vi "Set Camera Settings.vi"() -> ()   [LabVIEW 2020, in "examples.lvlib"]
uses:
  examples.lvlib
  6edc065a-5b9d-4876-ad44-0cda83ee0fad.vi
  capture/Stream/Stream.lvclass
  capture/capture.lvlib
  capture/Stream/Get Saturation Parameter Info.vi
  image/image.lvlib
  capture/Stream/Get Brightenss Parameter Info.vi
  capture/Stream/Get Brightenss Parameter.vi
  capture/Stream/Get Contrast Parameter Info.vi
  capture/Stream/Get Contrast Parameter.vi
  capture/Stream/Get Gain Parameter Info.vi
  capture/Stream/Get Powerline Frequency Parameter Info.vi
  capture/Stream/Get Gain Parameter.vi
  capture/Stream/Get Powerline Frequency Parameter.vi
  capture/Stream/Get Zoom Parameter.vi
  image/New Image (ARGB Preallocated).vi
  capture/Stream/Get Backlight Compensation Parameter.vi
  capture/Stream/Get Hue Parameter Info.vi
  capture/Stream/Get Hue Parameter.vi
  capture/Stream/Get Gamma Parameter Info.vi
  capture/Stream/Get Gamma Parameter.vi
  capture/Stream/Get Zoom Parameter Info.vi
  capture/Stream/Get White Balance Parameter Info.vi
  capture/Stream/Get Saturation Parameter.vi
  capture/Stream/Get White Balance Parameter.vi
  capture/Stream/Get Sharpness Parameter.vi
  capture/Stream/Get Focus Parameter Info.vi
  capture/Stream/Get Exposure Parameter Info.vi
  capture/Stream/Get Exposure Parameter.vi
  capture/Stream/Get Focus Parameter.vi
  capture/Stream/Get Backlight Compensation Parameter Info.vi
  capture/Stream/Set Powerline Frequency Parameter.vi
  capture/Stream/Set Hue Parameter.vi
  capture/Stream/Set White Balance Parameter.vi
  capture/Stream/Set Brightenss Parameter.vi
  capture/Stream/Set Zoom Parameter.vi
  capture/Stream/Set Contrast Parameter.vi
  capture/Stream/Set Gain Parameter.vi
  capture/Stream/Set Backlight Compensation Parameter.vi
  capture/Stream/Set Saturation Parameter.vi
  capture/Stream/Set Gamma Parameter.vi
  capture/Stream/Set Focus Parameter.vi
  capture/Stream/Set Sharpness Parameter.vi
  capture/Stream/Set Exposure Parameter.vi
  image/Draw Image to Picture (ARGB).vi
  dec5b208-33d2-3fcd-38b9-acb140bbe53f.vi
panel:
  in  "Hue":i32(slide) scale=-180.0..180.0
  in  "Gamma":i32(slide) scale=90.0..150.0
  in  "Zoom":i32(slide) scale=100.0..400.0
  in  "Whitebalance":i32(slide) scale=2800.0..6500.0
  in  "Sharpness":i32(slide) scale=0.0..100.0
  in  "Saturation":i32(slide) scale=0.0..100.0
  in  "Powerline Frequency":i32(slide) scale=-180.0..180.0
  in  "Gain":i32(slide) scale=0.0..2.0
  in  "Backlight Compensation":i32(slide) scale=0.0..2.0
  in  "Focus":i32(slide) scale=-11.0..-3.0
  in  "Exposure":i32(slide) scale=-11.0..-3.0
  in  "Contrast":i32(slide) scale=0.0..255.0
  in  "Brightness":i32(slide) scale=0.0..255.0
  out "2D Picture":picture
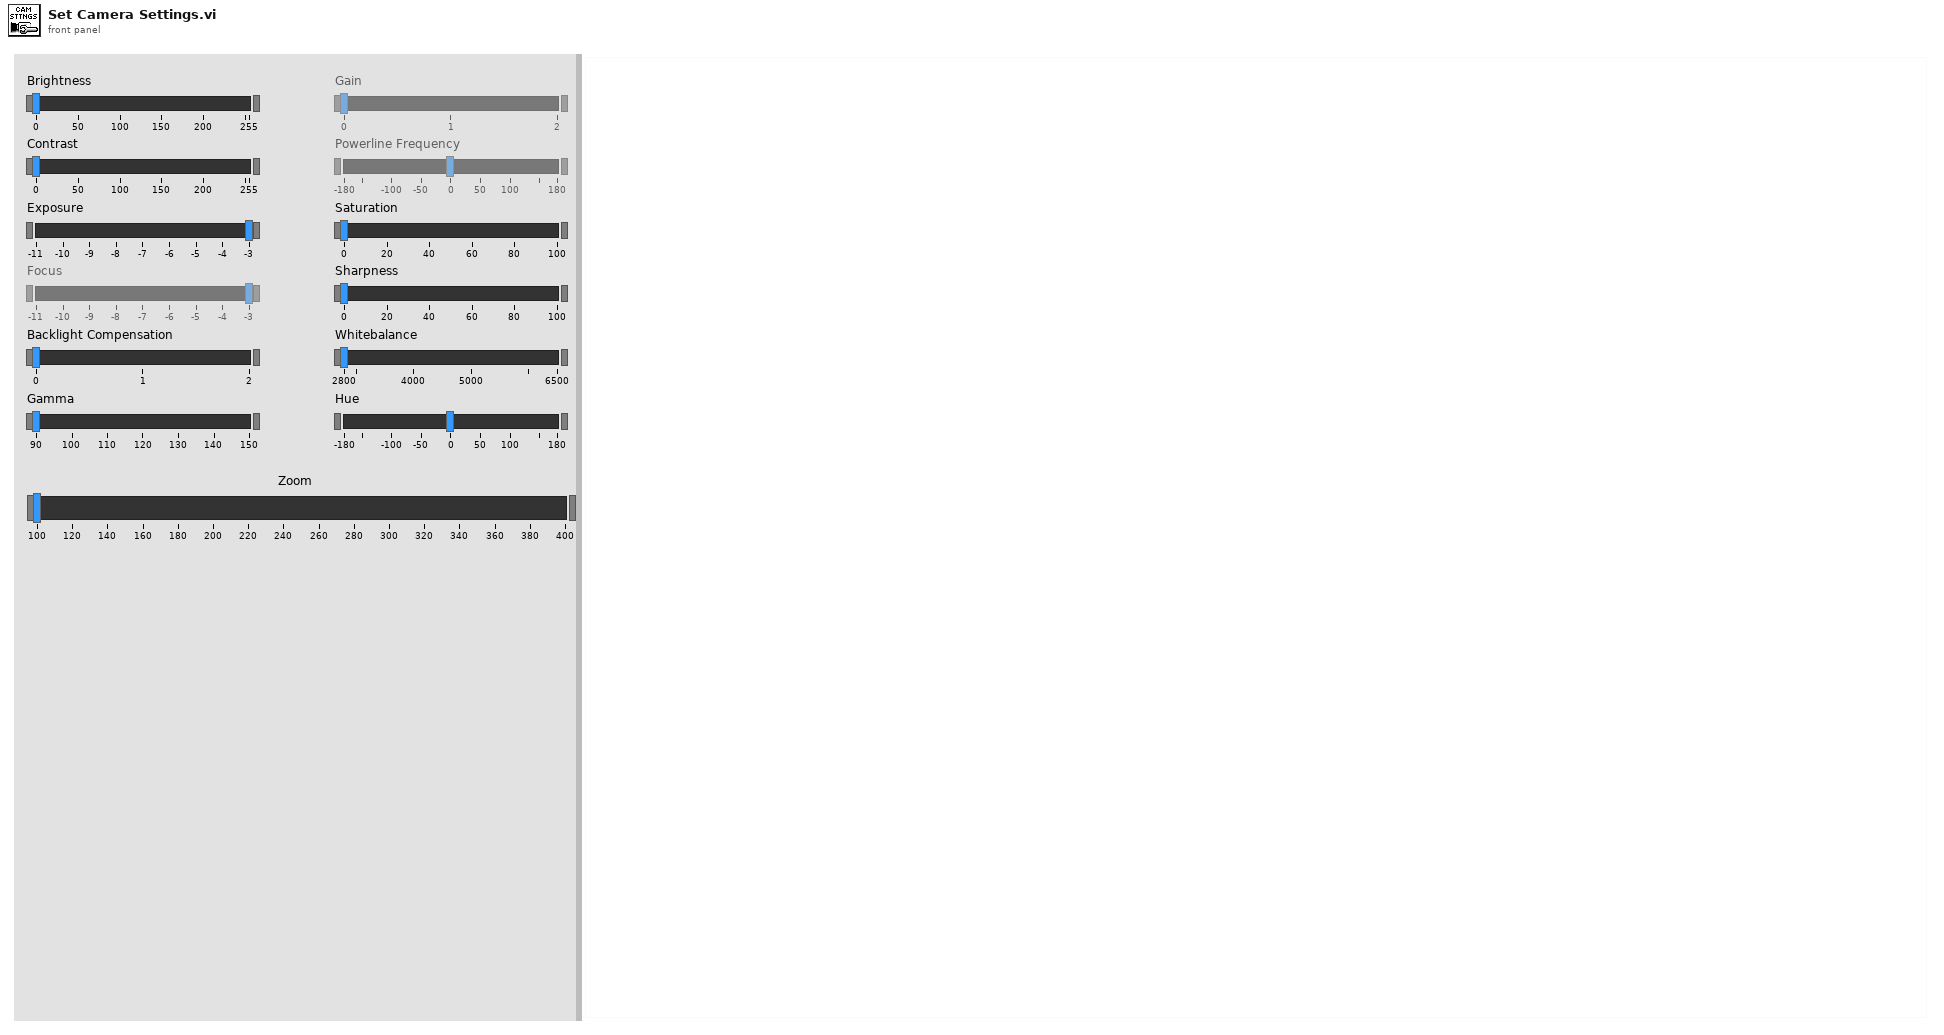
[diagram p1: front panel]
types:
  T1 = enum16{"Brightness", "Contrast", "Exposure", "Focus", "Backlight Compensation", "Gain", "Gamma", "Hue", "Powerline Frequency", "Saturation", "Sharpness", "Whitebalance", "Zoom"}
  T2 = typedef "capture.lvlib/Stream.lvclass/Stream Specification.ctl" = cluster{"Size":T3, "FPS":T4}
  T3 = typedef "common.lvlib/Image Size (Integer).ctl" = cluster{"Width":u16, "Height":u16}
  T4 = typedef "capture.lvlib/Stream.lvclass/Frames per Second.ctl" = cluster{"Numerator":u32, "Denominator":u32}
  T5 = cluster{"ID":string, "Name":string, "Stream Specifications":T2[]}[]
  T6 = cluster{"ID":string, "Name":string, "Stream Specifications":T2[]}
  T7 = enum16{"Brightness", "Contrast", "Exposure", "Focus", "Backlight Compensation", "Gain", "Gamma", "Hue", "Powerline Frequency", "Saturation", "Sharpness", "Whitebalance", "Zoom"}[]
  T8 = enum8{"Enabled", "Disabled", "Disabled and Grayed Out"}
  T9 = typedef "capture.lvlib/Stream.lvclass/Camera Parameter Information.ctl" = cluster{"Is Supported":bool, "Max":i32, "Min":i32, "Step":i32, "Default":i32}
  T10 = typedef "image.lvlib/ARGB Image.ctl" = refnum<data-value>
  T11 = typedef "image.lvlib/Image Draw Offset.ctl" = cluster{"Left":i16, "Top":i16}
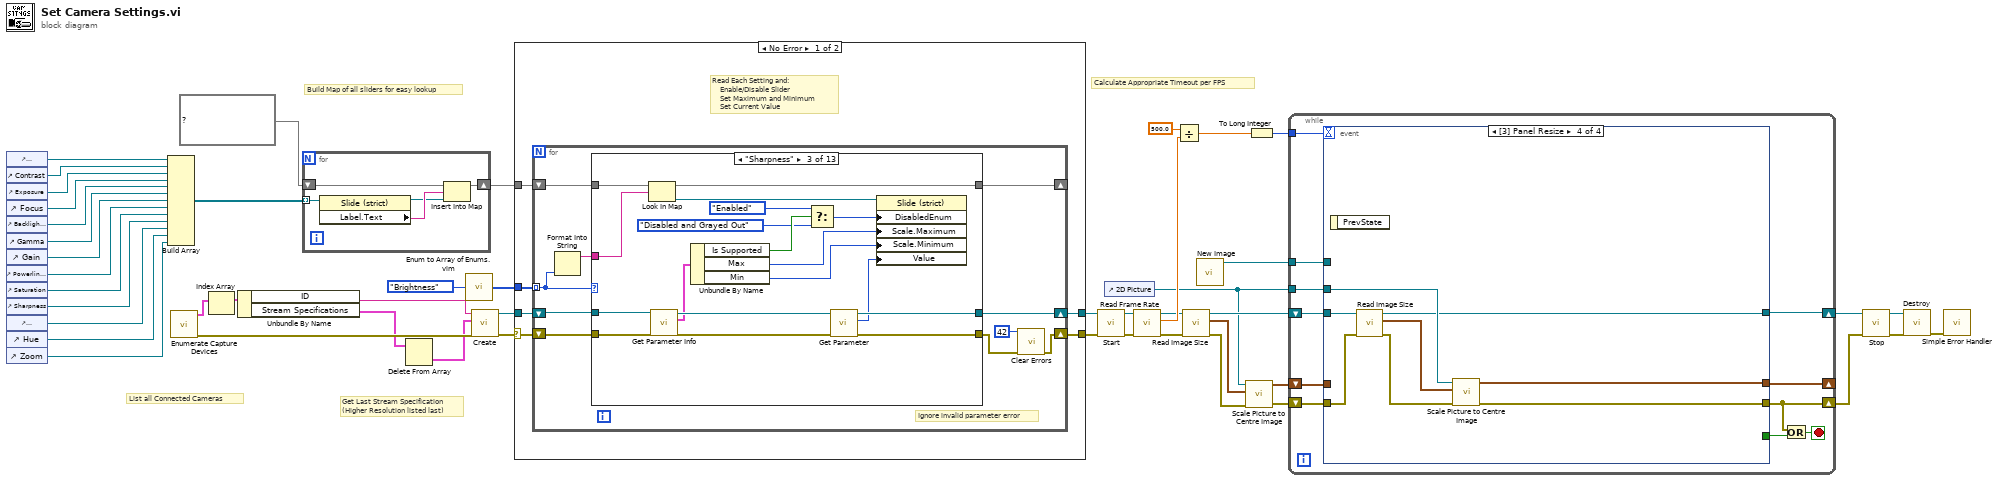
[diagram p0: block diagram]
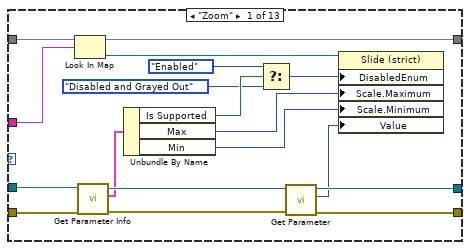
[diagram p2: hidden frame]
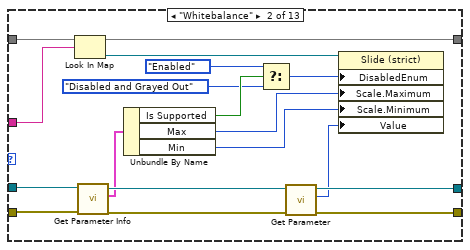
[diagram p3: hidden frame]
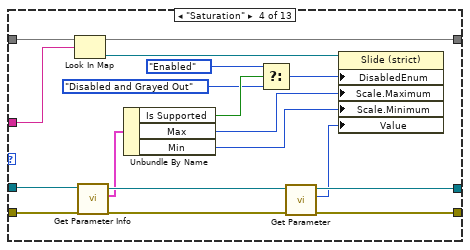
[diagram p4: hidden frame]
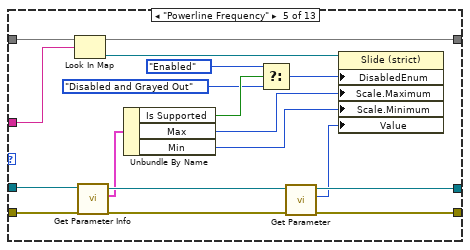
[diagram p5: hidden frame]
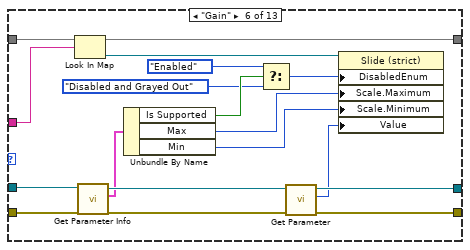
[diagram p6: hidden frame]
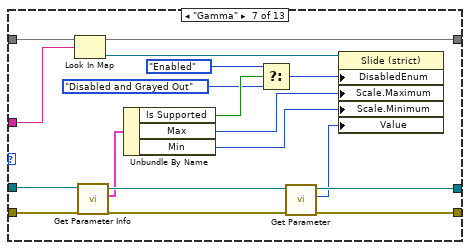
[diagram p7: hidden frame]
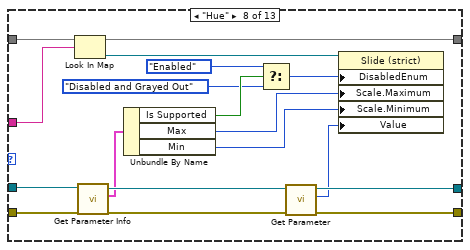
[diagram p8: hidden frame]
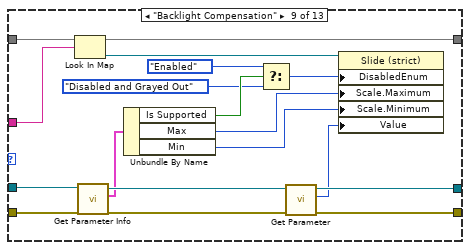
[diagram p9: hidden frame]
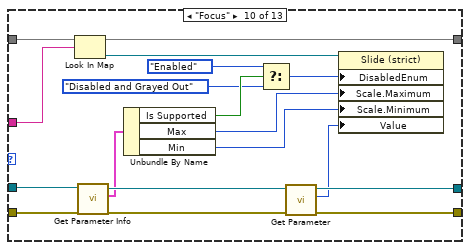
[diagram p10: hidden frame]
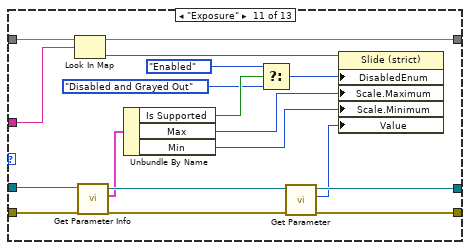
[diagram p11: hidden frame]
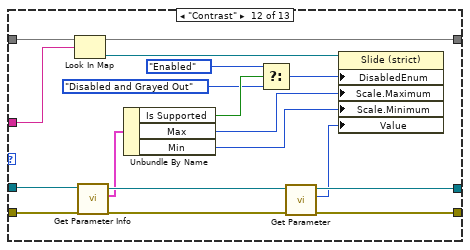
[diagram p12: hidden frame]
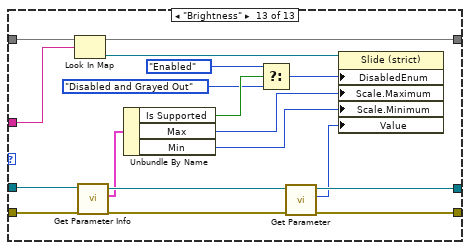
[diagram p13: hidden frame]
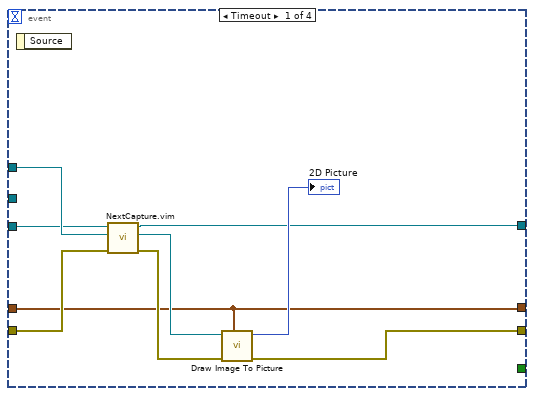
[diagram p15: hidden frame]
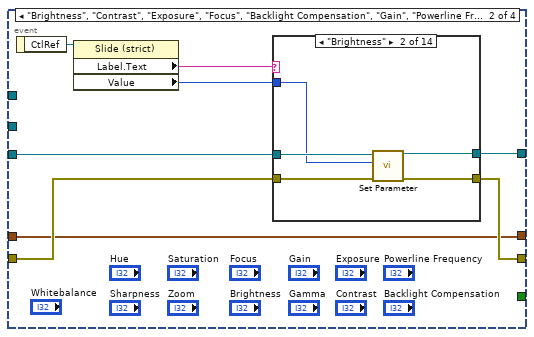
[diagram p16: hidden frame]
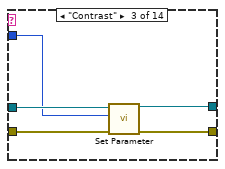
[diagram p18: hidden frame]
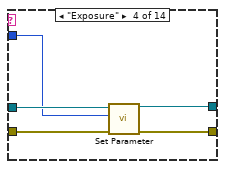
[diagram p19: hidden frame]
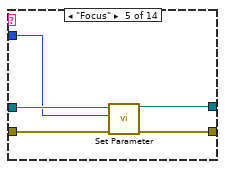
[diagram p20: hidden frame]
diagram:
  # "Calculate Appropriate Timeout per FPS"
  # "Build Map of all sliders for easy lookup"
  # "Get Last Stream Specification\n(Higher Resolution listed last)"
  # "List all Connected Cameras"
  n1 = control-ref of="Brightness"() -> (w40:refnum<vi>)
  n2 = control-ref of="Contrast"() -> (w39:refnum<vi>)
  n3 = control-ref of="Exposure"() -> (w38:refnum<vi>)
  n4 = control-ref of="Focus"() -> (w37:refnum<vi>)
  n5 = control-ref of="Backlight Compensation"() -> (w36:refnum<vi>)
  n6 = control-ref of="Gamma"() -> (w35:refnum<vi>)
  n7 = control-ref of="Gain"() -> (w34:refnum<vi>)
  n8 = control-ref of="Powerline Frequency"() -> (w33:refnum<vi>)
  n9 = control-ref of="Saturation"() -> (w32:refnum<vi>)
  n10 = control-ref of="Sharpness"() -> (w31:refnum<vi>)
  n11 = control-ref of="Whitebalance"() -> (w30:refnum<vi>)
  n12 = control-ref of="Hue"() -> (w29:refnum<vi>)
  n13 = control-ref of="Zoom"() -> (w28:refnum<vi>)
  n14 = Build Array(w40, w39, w38, w37, w36, w35, w34, w33, w32, w31, w30, w29, w28) -> (w27:refnum<vi>[])
  n15 = call "Enumerate Capture Devices.vi"() -> ("error out"=w42:errorcluster, "Devices"=w45:T5)  [unwired: 10 in]
  n16 = Index Array(array=w45) -> (element=w44:T6)  [unwired: 1 in]
  n17 = Unbundle By Name(w44) -> ("ID"=w43:string, "Stream Specifications"=w10:T2[])
  n18 = for {
    tunnel: w27 -> [w53] mode=indexing
    shift-right: [w49] -> w25
    shift-left: map{string, refnum<vi>} {} ("map in") -> [w50]
    n19 = property class="Slide (strict)"(reference=w53) -> (reference out=w51:refnum<vi>, "Label.Text"=w52:string)  [unwired: 1 in, 1 out]
    n20 = Insert Into Map(map in=w50, key=w52, value=w51) -> (map out=w49:map{string, refnum<vi>})  [unwired: 2 out]
  }
  n21 = Delete From Array(array=w10) -> (deleted portion=w41:T2)  [unwired: 2 in, 1 out]
  n22 = call "Enum to Array of Enums.vim"("enum"=T1."Brightness") -> ("array of enums"=w47:T7)
  n23 = call "Create.vi"("error in (no error)"=w42, "Desired Stream Specification"=w41, "Device ID"=w43) -> ("error out"=w9:errorcluster, "Stream"=w46:refnum<class "Stream.lvclass">)  [unwired: 7 in]
  n24 = case shown="No Error" w9 {
    selector: w9 -> [w55 w291]
    tunnel: w47 -> [w59 _]
    tunnel: w46 -> [w58 w292]
    tunnel: w25 -> [w57 _]
    tunnel: [w56 w292] -> w21
    tunnel: [w54 w291] -> w8
    frame No Error {
      # "Read Each Setting and:\n    Enable/Disable Slider\n    Set Maximum and Minimum\n    Set Current Value"
      n25 = for {
        tunnel: w59 -> [w61] mode=indexing
        shift-right: [w68] -> w56
        shift-left: w58 -> [w69]
        shift-right: [w66] -> _
        shift-left: w57 -> [w67]
        shift-right: [w62] -> w54
        shift-left: w55 -> [w65]
        # "Ignore invalid parameter error"
        n26 = Format Into String(w61) -> (resulting string=w60:string)  [unwired: 3 in, 1 out]
        n27 = case shown="\"Sharpness\"" w61 {
          tunnel: w69 -> [w86 w103 w120 w137 w154 w171 w188 w205 w222 w239 w256 w273 w290]
          tunnel: [w84 w100 w117 w134 w151 w168 w185 w202 w219 w236 w253 w270 w287] -> w68
          tunnel: w67 -> [w74 w90 w107 w124 w141 w158 w175 w192 w209 w226 w243 w260 w277]
          tunnel: [w74 w90 w107 w124 w141 w158 w175 w192 w209 w226 w243 w260 w277] -> w66
          tunnel: w65 -> [w73 w89 w106 w123 w140 w157 w174 w191 w208 w225 w242 w259 w276]
          tunnel: [w71 w88 w105 w122 w139 w156 w173 w190 w207 w224 w241 w258 w275] -> w63
          tunnel: w60 -> [w70 w87 w104 w121 w138 w155 w172 w189 w206 w223 w240 w257 w274]
          frame "Zoom" {
            n28 = Look In Map(map=w74, key=w70) -> (value=w83:refnum<vi>)  [unwired: 1 in, 1 out]
            n29 = call-poly "Get Parameter Info.vi"("error in (no error)"=w73, "Stream in"=w86) -> ("error out"=w72:errorcluster, "Info"=w81:T9, "Stream"=w85:refnum<class "Stream.lvclass">)  [unwired: 7 in]
            n30 = Unbundle By Name(w81) -> ("Is Supported"=w78:bool, "Max"=w80:i32, "Min"=w79:i32)
            n31 = Select(t=T8."Enabled" ("Disabled"), s=w78, f=T8."Disabled and Grayed Out" ("Disabled")) -> (s? t:f=w76:T8)
            n32 = call-poly "Get Parameter.vi"("error in (no error)"=w72, "Stream in"=w85) -> ("error out"=w71:errorcluster, "Value"=w82:i32, "Stream"=w84:refnum<class "Stream.lvclass">)  [unwired: 7 in]
            n33 = property on="Property Node" class="Slide (strict)"(reference=w83, "DisabledEnum"=w76, "Scale.Maximum"=w80, "Scale.Minimum"=w79, "Value"=w82) -> ()  [unwired: 1 in, 2 out]
          }
          frame "Whitebalance" {
            n34 = Look In Map(map=w90, key=w87) -> (value=w99:refnum<vi>)  [unwired: 1 in, 1 out]
            n35 = call-poly "Get Parameter Info.vi"("error in (no error)"=w89, "Stream in"=w103) -> ("error out"=w101:errorcluster, "Info"=w97:T9, "Stream"=w102:refnum<class "Stream.lvclass">)  [unwired: 7 in]
            n36 = Unbundle By Name(w97) -> ("Is Supported"=w94:bool, "Max"=w96:i32, "Min"=w95:i32)
            n37 = Select(t=T8."Enabled" ("Disabled"), s=w94, f=T8."Disabled and Grayed Out" ("Disabled")) -> (s? t:f=w92:T8)
            n38 = call-poly "Get Parameter.vi"("error in (no error)"=w101, "Stream in"=w102) -> ("error out"=w88:errorcluster, "Value"=w98:i32, "Stream"=w100:refnum<class "Stream.lvclass">)  [unwired: 7 in]
            n39 = property on="Property Node" class="Slide (strict)"(reference=w99, "DisabledEnum"=w92, "Scale.Maximum"=w96, "Scale.Minimum"=w95, "Value"=w98) -> ()  [unwired: 1 in, 2 out]
          }
          frame "Sharpness" {
            n40 = Look In Map(map=w107, key=w104) -> (value=w116:refnum<vi>)  [unwired: 1 in, 1 out]
            n41 = call-poly "Get Parameter Info.vi"("error in (no error)"=w106, "Stream in"=w120) -> ("error out"=w118:errorcluster, "Info"=w114:T9, "Stream"=w119:refnum<class "Stream.lvclass">)  [unwired: 7 in]
            n42 = Unbundle By Name(w114) -> ("Is Supported"=w111:bool, "Max"=w113:i32, "Min"=w112:i32)
            n43 = Select(t=T8."Enabled" ("Disabled"), s=w111, f=T8."Disabled and Grayed Out" ("Disabled")) -> (s? t:f=w109:T8)
            n44 = call-poly "Get Parameter.vi"("error in (no error)"=w118, "Stream in"=w119) -> ("error out"=w105:errorcluster, "Value"=w115:i32, "Stream"=w117:refnum<class "Stream.lvclass">)  [unwired: 7 in]
            n45 = property on="Property Node" class="Slide (strict)"(reference=w116, "DisabledEnum"=w109, "Scale.Maximum"=w113, "Scale.Minimum"=w112, "Value"=w115) -> ()  [unwired: 1 in, 2 out]
          }
          frame "Saturation" {
            n46 = Look In Map(map=w124, key=w121) -> (value=w133:refnum<vi>)  [unwired: 1 in, 1 out]
            n47 = call-poly "Get Parameter Info.vi"("error in (no error)"=w123, "Stream in"=w137) -> ("error out"=w135:errorcluster, "Info"=w131:T9, "Stream"=w136:refnum<class "Stream.lvclass">)  [unwired: 7 in]
            n48 = Unbundle By Name(w131) -> ("Is Supported"=w128:bool, "Max"=w130:i32, "Min"=w129:i32)
            n49 = Select(t=T8."Enabled" ("Disabled"), s=w128, f=T8."Disabled and Grayed Out" ("Disabled")) -> (s? t:f=w126:T8)
            n50 = call-poly "Get Parameter.vi"("error in (no error)"=w135, "Stream in"=w136) -> ("error out"=w122:errorcluster, "Value"=w132:i32, "Stream"=w134:refnum<class "Stream.lvclass">)  [unwired: 7 in]
            n51 = property on="Property Node" class="Slide (strict)"(reference=w133, "DisabledEnum"=w126, "Scale.Maximum"=w130, "Scale.Minimum"=w129, "Value"=w132) -> ()  [unwired: 1 in, 2 out]
          }
          frame "Powerline Frequency" {
            n52 = Look In Map(map=w141, key=w138) -> (value=w150:refnum<vi>)  [unwired: 1 in, 1 out]
            n53 = call-poly "Get Parameter Info.vi"("error in (no error)"=w140, "Stream in"=w154) -> ("error out"=w152:errorcluster, "Info"=w148:T9, "Stream"=w153:refnum<class "Stream.lvclass">)  [unwired: 7 in]
            n54 = Unbundle By Name(w148) -> ("Is Supported"=w145:bool, "Max"=w147:i32, "Min"=w146:i32)
            n55 = Select(t=T8."Enabled" ("Disabled"), s=w145, f=T8."Disabled and Grayed Out" ("Disabled")) -> (s? t:f=w143:T8)
            n56 = call-poly "Get Parameter.vi"("error in (no error)"=w152, "Stream in"=w153) -> ("error out"=w139:errorcluster, "Value"=w149:i32, "Stream"=w151:refnum<class "Stream.lvclass">)  [unwired: 7 in]
            n57 = property on="Property Node" class="Slide (strict)"(reference=w150, "DisabledEnum"=w143, "Scale.Maximum"=w147, "Scale.Minimum"=w146, "Value"=w149) -> ()  [unwired: 1 in, 2 out]
          }
          frame "Gain" {
            n58 = Look In Map(map=w158, key=w155) -> (value=w167:refnum<vi>)  [unwired: 1 in, 1 out]
            n59 = call-poly "Get Parameter Info.vi"("error in (no error)"=w157, "Stream in"=w171) -> ("error out"=w169:errorcluster, "Info"=w165:T9, "Stream"=w170:refnum<class "Stream.lvclass">)  [unwired: 7 in]
            n60 = Unbundle By Name(w165) -> ("Is Supported"=w162:bool, "Max"=w164:i32, "Min"=w163:i32)
            n61 = Select(t=T8."Enabled" ("Disabled"), s=w162, f=T8."Disabled and Grayed Out" ("Disabled")) -> (s? t:f=w160:T8)
            n62 = call-poly "Get Parameter.vi"("error in (no error)"=w169, "Stream in"=w170) -> ("error out"=w156:errorcluster, "Value"=w166:i32, "Stream"=w168:refnum<class "Stream.lvclass">)  [unwired: 7 in]
            n63 = property on="Property Node" class="Slide (strict)"(reference=w167, "DisabledEnum"=w160, "Scale.Maximum"=w164, "Scale.Minimum"=w163, "Value"=w166) -> ()  [unwired: 1 in, 2 out]
          }
          frame "Gamma" {
            n64 = Look In Map(map=w175, key=w172) -> (value=w184:refnum<vi>)  [unwired: 1 in, 1 out]
            n65 = call-poly "Get Parameter Info.vi"("error in (no error)"=w174, "Stream in"=w188) -> ("error out"=w186:errorcluster, "Info"=w182:T9, "Stream"=w187:refnum<class "Stream.lvclass">)  [unwired: 7 in]
            n66 = Unbundle By Name(w182) -> ("Is Supported"=w179:bool, "Max"=w181:i32, "Min"=w180:i32)
            n67 = Select(t=T8."Enabled" ("Disabled"), s=w179, f=T8."Disabled and Grayed Out" ("Disabled")) -> (s? t:f=w177:T8)
            n68 = call-poly "Get Parameter.vi"("error in (no error)"=w186, "Stream in"=w187) -> ("error out"=w173:errorcluster, "Value"=w183:i32, "Stream"=w185:refnum<class "Stream.lvclass">)  [unwired: 7 in]
            n69 = property on="Property Node" class="Slide (strict)"(reference=w184, "DisabledEnum"=w177, "Scale.Maximum"=w181, "Scale.Minimum"=w180, "Value"=w183) -> ()  [unwired: 1 in, 2 out]
          }
          frame "Hue" {
            n70 = Look In Map(map=w192, key=w189) -> (value=w201:refnum<vi>)  [unwired: 1 in, 1 out]
            n71 = call-poly "Get Parameter Info.vi"("error in (no error)"=w191, "Stream in"=w205) -> ("error out"=w203:errorcluster, "Info"=w199:T9, "Stream"=w204:refnum<class "Stream.lvclass">)  [unwired: 7 in]
            n72 = Unbundle By Name(w199) -> ("Is Supported"=w196:bool, "Max"=w198:i32, "Min"=w197:i32)
            n73 = Select(t=T8."Enabled" ("Disabled"), s=w196, f=T8."Disabled and Grayed Out" ("Disabled")) -> (s? t:f=w194:T8)
            n74 = call-poly "Get Parameter.vi"("error in (no error)"=w203, "Stream in"=w204) -> ("error out"=w190:errorcluster, "Value"=w200:i32, "Stream"=w202:refnum<class "Stream.lvclass">)  [unwired: 7 in]
            n75 = property on="Property Node" class="Slide (strict)"(reference=w201, "DisabledEnum"=w194, "Scale.Maximum"=w198, "Scale.Minimum"=w197, "Value"=w200) -> ()  [unwired: 1 in, 2 out]
          }
          frame "Backlight Compensation" {
            n76 = Look In Map(map=w209, key=w206) -> (value=w218:refnum<vi>)  [unwired: 1 in, 1 out]
            n77 = call-poly "Get Parameter Info.vi"("error in (no error)"=w208, "Stream in"=w222) -> ("error out"=w220:errorcluster, "Info"=w216:T9, "Stream"=w221:refnum<class "Stream.lvclass">)  [unwired: 7 in]
            n78 = Unbundle By Name(w216) -> ("Is Supported"=w213:bool, "Max"=w215:i32, "Min"=w214:i32)
            n79 = Select(t=T8."Enabled" ("Disabled"), s=w213, f=T8."Disabled and Grayed Out" ("Disabled")) -> (s? t:f=w211:T8)
            n80 = call-poly "Get Parameter.vi"("error in (no error)"=w220, "Stream in"=w221) -> ("error out"=w207:errorcluster, "Value"=w217:i32, "Stream"=w219:refnum<class "Stream.lvclass">)  [unwired: 7 in]
            n81 = property on="Property Node" class="Slide (strict)"(reference=w218, "DisabledEnum"=w211, "Scale.Maximum"=w215, "Scale.Minimum"=w214, "Value"=w217) -> ()  [unwired: 1 in, 2 out]
          }
          frame "Focus" {
            n82 = Look In Map(map=w226, key=w223) -> (value=w235:refnum<vi>)  [unwired: 1 in, 1 out]
            n83 = call-poly "Get Parameter Info.vi"("error in (no error)"=w225, "Stream in"=w239) -> ("error out"=w237:errorcluster, "Info"=w233:T9, "Stream"=w238:refnum<class "Stream.lvclass">)  [unwired: 7 in]
            n84 = Unbundle By Name(w233) -> ("Is Supported"=w230:bool, "Max"=w232:i32, "Min"=w231:i32)
            n85 = Select(t=T8."Enabled" ("Disabled"), s=w230, f=T8."Disabled and Grayed Out" ("Disabled")) -> (s? t:f=w228:T8)
            n86 = call-poly "Get Parameter.vi"("error in (no error)"=w237, "Stream in"=w238) -> ("error out"=w224:errorcluster, "Value"=w234:i32, "Stream"=w236:refnum<class "Stream.lvclass">)  [unwired: 7 in]
            n87 = property on="Property Node" class="Slide (strict)"(reference=w235, "DisabledEnum"=w228, "Scale.Maximum"=w232, "Scale.Minimum"=w231, "Value"=w234) -> ()  [unwired: 1 in, 2 out]
          }
          frame "Exposure" {
            n88 = Look In Map(map=w243, key=w240) -> (value=w252:refnum<vi>)  [unwired: 1 in, 1 out]
            n89 = call-poly "Get Parameter Info.vi"("error in (no error)"=w242, "Stream in"=w256) -> ("error out"=w254:errorcluster, "Info"=w250:T9, "Stream"=w255:refnum<class "Stream.lvclass">)  [unwired: 7 in]
            n90 = Unbundle By Name(w250) -> ("Is Supported"=w247:bool, "Max"=w249:i32, "Min"=w248:i32)
            n91 = Select(t=T8."Enabled" ("Disabled"), s=w247, f=T8."Disabled and Grayed Out" ("Disabled")) -> (s? t:f=w245:T8)
            n92 = call-poly "Get Parameter.vi"("error in (no error)"=w254, "Stream in"=w255) -> ("error out"=w241:errorcluster, "Value"=w251:i32, "Stream"=w253:refnum<class "Stream.lvclass">)  [unwired: 7 in]
            n93 = property on="Property Node" class="Slide (strict)"(reference=w252, "DisabledEnum"=w245, "Scale.Maximum"=w249, "Scale.Minimum"=w248, "Value"=w251) -> ()  [unwired: 1 in, 2 out]
          }
          frame "Contrast" {
            n94 = Look In Map(map=w260, key=w257) -> (value=w269:refnum<vi>)  [unwired: 1 in, 1 out]
            n95 = call-poly "Get Parameter Info.vi"("error in (no error)"=w259, "Stream in"=w273) -> ("error out"=w271:errorcluster, "Info"=w267:T9, "Stream"=w272:refnum<class "Stream.lvclass">)  [unwired: 7 in]
            n96 = Unbundle By Name(w267) -> ("Is Supported"=w264:bool, "Max"=w266:i32, "Min"=w265:i32)
            n97 = Select(t=T8."Enabled" ("Disabled"), s=w264, f=T8."Disabled and Grayed Out" ("Disabled")) -> (s? t:f=w262:T8)
            n98 = call-poly "Get Parameter.vi"("error in (no error)"=w271, "Stream in"=w272) -> ("error out"=w258:errorcluster, "Value"=w268:i32, "Stream"=w270:refnum<class "Stream.lvclass">)  [unwired: 7 in]
            n99 = property on="Property Node" class="Slide (strict)"(reference=w269, "DisabledEnum"=w262, "Scale.Maximum"=w266, "Scale.Minimum"=w265, "Value"=w268) -> ()  [unwired: 1 in, 2 out]
          }
          frame "Brightness" {
            n100 = Look In Map(map=w277, key=w274) -> (value=w286:refnum<vi>)  [unwired: 1 in, 1 out]
            n101 = call-poly "Get Parameter Info.vi"("error in (no error)"=w276, "Stream in"=w290) -> ("error out"=w288:errorcluster, "Info"=w284:T9, "Stream"=w289:refnum<class "Stream.lvclass">)  [unwired: 7 in]
            n102 = Unbundle By Name(w284) -> ("Is Supported"=w281:bool, "Max"=w283:i32, "Min"=w282:i32)
            n103 = Select(t=T8."Enabled" ("Disabled"), s=w281, f=T8."Disabled and Grayed Out" ("Disabled")) -> (s? t:f=w279:T8)
            n104 = call-poly "Get Parameter.vi"("error in (no error)"=w288, "Stream in"=w289) -> ("error out"=w275:errorcluster, "Value"=w285:i32, "Stream"=w287:refnum<class "Stream.lvclass">)  [unwired: 7 in]
            n105 = property on="Property Node" class="Slide (strict)"(reference=w286, "DisabledEnum"=w279, "Scale.Maximum"=w283, "Scale.Minimum"=w282, "Value"=w285) -> ()  [unwired: 1 in, 2 out]
          }
        }
        n106 = call <vilib>:"Clear Errors.vi"("error in (no error)"=w63, "specific error code to clear (0: all)"=42) -> ("error out"=w62:errorcluster)  [unwired: 4 in, 1 out]
      }
    }
    frame Error {
    }
  }
  n107 = call "Start.vi"("error in (no error)"=w8, "Stream in"=w21) -> ("error out"=w19:errorcluster, "Stream"=w20:refnum<class "Stream.lvclass">)  [unwired: 8 in]
  n108 = control-ref of="2D Picture"() -> (w1:refnum<vi>)
  n109 = call "Read Frame Rate.vi"("error in (no error)"=w19, "Stream in"=w20) -> ("error out"=w16:errorcluster, "Frame Rate (FPS)"=w24:dbl, "Stream"=w7:refnum<class "Stream.lvclass">)  [unwired: 7 in]
  n110 = Divide(x=500.0, y=w24) -> (x/y=w23:dbl)
  n111 = call "Read Image Size.vi"("error in (no error)"=w16, "Stream in"=w7) -> ("error out"=w4:errorcluster, "Image Size"=w5:T3, "Stream"=w6:refnum<class "Stream.lvclass">)  [unwired: 7 in]
  n112 = call-poly "New Image.vi"() -> ("ARGB Image"=w17:T10)  [unwired: 10 in, 1 out]
  n113 = call "Scale Picture to Centre Image.vi"("error in (no error)"=w4, "Image Size"=w5, "Picture in"=w1) -> ("error out"=w3:errorcluster, "Draw Image to Picture Offset"=w2:T11)  [unwired: 6 in, 1 out]
  n114 = To Long Integer(number=w23) -> (32bit integer=w18:i32)
  n115 = while {
    tunnel: w18 -> [w303]
    tunnel: w17 -> [w302]
    shift-right: [w297] -> w15
    shift-left: w3 -> [w300]
    shift-right: [w296] -> w14
    shift-left: w6 -> [w301]
    tunnel: w1 -> [w294]
    shift-right: [w293] -> _
    shift-left: w2 -> [w295]
    stop <- w299 stop-if-true
    n116 = event shown="[3] Panel Resize" {
      selector: _ -> [_ _ _ _]
      dyn-events: _ -> [_ _ _ _]
      timeout: w303 -> [_ _ _ _]
      tunnel: w302 -> [w310 _ w391 _]
      tunnel: w301 -> [w309 w318 w389 w400]
      tunnel: w300 -> [w308 w317 w390 w399]
      tunnel: [w306 w320 w390 w396] -> w297
      tunnel: [_ _ w392 _] -> w298
      tunnel: [w305 w319 w389 w394] -> w296
      tunnel: w295 -> [w304 w313 w388 _]
      tunnel: w294 -> [_ _ _ w397]
      tunnel: [w304 w313 w388 w393] -> w293
      event Timeout {
        n117 = event-data() -> ()  [unwired: 1 in, 1 out]
        n118 = call "NextCapture.vim"("error in (no error)"=w308, "ARGB Image Destination in"=w310, "Stream in"=w309) -> ("error out"=w307:errorcluster, "ARGB Image"=w312:T10, "Stream"=w305:refnum<class "Stream.lvclass">)  [unwired: 5 in, 1 out]
        n119 = call-poly "Draw Image To Picture.vi"("Image Draw Offset (Default 0,0)"=w304, "error in (no error)"=w307, "ARGB Image Source in"=w312) -> ("error out"=w306:errorcluster, "Picture"=→"2D Picture":picture)  [unwired: 7 in]
      }
      event "Brightness", "Contrast", "Exposure", "Focus", "Backlight Compensation", "Gain", "Powerline Frequency", "Saturation", "Sharpness", "Whitebalance", "Zoom", "Gamma", "Hue": Value Change {
        n120 = event-data() -> ("CtlRef"=w316:refnum<vi>)  [unwired: 1 in]
        n121 = property class="Slide (strict)"(reference=w316) -> ("Label.Text"=w315:string, "Value"=w314:i32)  [unwired: 1 in, 2 out]
        n122 = case shown="\"Brightness\"" w315 {
          tunnel: [w321 w327 w332 w337 w342 w347 w352 w357 w362 w367 w372 w377 w382 w387] -> w320
          tunnel: [w322 w326 w331 w336 w341 w346 w351 w356 w361 w366 w371 w376 w381 w386] -> w319
          tunnel: w318 -> [w322 w325 w330 w335 w340 w345 w350 w355 w360 w365 w370 w375 w380 w385]
          tunnel: w317 -> [w321 w324 w329 w334 w339 w344 w349 w354 w359 w364 w369 w374 w379 w384]
          tunnel: w314 -> [_ w323 w328 w333 w338 w343 w348 w353 w358 w363 w368 w373 w378 w383]
          frame Default {
          }
          frame "Brightness" {
            n123 = call-poly "Set Parameter.vi"("error in (no error)"=w324, "Value"=w323, "Stream in"=w325) -> ("error out"=w327:errorcluster, "Stream"=w326:refnum<class "Stream.lvclass">)  [unwired: 6 in, 1 out]
          }
          frame "Contrast" {
            n124 = call-poly "Set Parameter.vi"("error in (no error)"=w329, "Value"=w328, "Stream in"=w330) -> ("error out"=w332:errorcluster, "Stream"=w331:refnum<class "Stream.lvclass">)  [unwired: 6 in, 1 out]
          }
          frame "Exposure" {
            n125 = call-poly "Set Parameter.vi"("error in (no error)"=w334, "Value"=w333, "Stream in"=w335) -> ("error out"=w337:errorcluster, "Stream"=w336:refnum<class "Stream.lvclass">)  [unwired: 6 in, 1 out]
          }
          frame "Focus" {
            n126 = call-poly "Set Parameter.vi"("error in (no error)"=w339, "Value"=w338, "Stream in"=w340) -> ("error out"=w342:errorcluster, "Stream"=w341:refnum<class "Stream.lvclass">)  [unwired: 6 in, 1 out]
          }
          frame "Backlight Compensation" {
            n127 = call-poly "Set Parameter.vi"("error in (no error)"=w344, "Value"=w343, "Stream in"=w345) -> ("error out"=w347:errorcluster, "Stream"=w346:refnum<class "Stream.lvclass">)  [unwired: 6 in, 1 out]
          }
          frame "Gamma" {
            n128 = call-poly "Set Parameter.vi"("error in (no error)"=w349, "Value"=w348, "Stream in"=w350) -> ("error out"=w352:errorcluster, "Stream"=w351:refnum<class "Stream.lvclass">)  [unwired: 6 in, 1 out]
          }
          frame "Gain" {
            n129 = call-poly "Set Parameter.vi"("error in (no error)"=w354, "Value"=w353, "Stream in"=w355) -> ("error out"=w357:errorcluster, "Stream"=w356:refnum<class "Stream.lvclass">)  [unwired: 6 in, 1 out]
          }
          frame "Powerline Frequency" {
            n130 = call-poly "Set Parameter.vi"("error in (no error)"=w359, "Value"=w358, "Stream in"=w360) -> ("error out"=w362:errorcluster, "Stream"=w361:refnum<class "Stream.lvclass">)  [unwired: 6 in, 1 out]
          }
          frame "Saturation" {
            n131 = call-poly "Set Parameter.vi"("error in (no error)"=w364, "Value"=w363, "Stream in"=w365) -> ("error out"=w367:errorcluster, "Stream"=w366:refnum<class "Stream.lvclass">)  [unwired: 6 in, 1 out]
          }
          frame "Sharpness" {
            n132 = call-poly "Set Parameter.vi"("error in (no error)"=w369, "Value"=w368, "Stream in"=w370) -> ("error out"=w372:errorcluster, "Stream"=w371:refnum<class "Stream.lvclass">)  [unwired: 6 in, 1 out]
          }
          frame "Whitebalance" {
            n133 = call-poly "Set Parameter.vi"("error in (no error)"=w374, "Value"=w373, "Stream in"=w375) -> ("error out"=w377:errorcluster, "Stream"=w376:refnum<class "Stream.lvclass">)  [unwired: 6 in, 1 out]
          }
          frame "Hue" {
            n134 = call-poly "Set Parameter.vi"("error in (no error)"=w379, "Value"=w378, "Stream in"=w380) -> ("error out"=w382:errorcluster, "Stream"=w381:refnum<class "Stream.lvclass">)  [unwired: 6 in, 1 out]
          }
          frame "Zoom" {
            n135 = call-poly "Set Parameter.vi"("error in (no error)"=w384, "Value"=w383, "Stream in"=w385) -> ("error out"=w387:errorcluster, "Stream"=w386:refnum<class "Stream.lvclass">)  [unwired: 6 in, 1 out]
          }
        }
      }
      event Panel Close? {
        w392 = TRUE
        n136 = event-data() -> ()  [unwired: 1 in, 4 out]
        n137 = Delete Data Value Reference(data value reference=w391) -> ()  [unwired: 1 in, 2 out]
        n138 = event-data("Discard?"=w392) -> ()  [unwired: 1 in, 1 out]
      }
      event Panel Resize {
        n139 = event-data() -> ()  [unwired: 1 in, 1 out]
        n140 = call "Read Image Size.vi"("error in (no error)"=w399, "Stream in"=w400) -> ("error out"=w398:errorcluster, "Image Size"=w395:T3, "Stream"=w394:refnum<class "Stream.lvclass">)  [unwired: 7 in]
        n141 = call "Scale Picture to Centre Image.vi"("error in (no error)"=w398, "Image Size"=w395, "Picture in"=w397) -> ("error out"=w396:errorcluster, "Draw Image to Picture Offset"=w393:T11)  [unwired: 6 in, 1 out]
      }
    }
    n142 = Or(x=w297, y=w298) -> (x .or. y?=w299:bool)
  }
  n143 = call "Stop.vi"("error in (no error)"=w15, "Stream in"=w14) -> ("error out"=w13:errorcluster, "Stream"=w12:refnum<class "Stream.lvclass">)  [unwired: 8 in]
  n144 = call "Destroy.vi"("error in (no error)"=w13, "Stream in"=w12) -> ("error out"=w11:errorcluster)  [unwired: 9 in]
  n145 = call <vilib>:"Simple Error Handler.vi"("error in (no error)"=w11) -> ()  [unwired: 4 in, 5 out]
